vi "Config Scan Voltage.vi"(0 "VISA resource name":refnum<visa-resource-name>, 1 "Coupling (0)":i32 min=0 max=3, 2 "Floor (0.001)":dbl=0.001 min=0.0003 max=15.0, 3 "Ceiling (15)":dbl=15.0 min=0.0003 max=15.0, 4 "Method (discrete)":enum16{"discrete", "log10", "log2", "linear"}(ring), 5 "Method Value (1)":dbl=1.0 min=-100.0 max=100.0 format="%#_6f", 7 "error in":errorcluster) -> (20 "VISA resource name out":refnum<visa-resource-name>, 27 "error out":errorcluster)   [LabVIEW 2019, in "Andeen-Hagerling 2700(400 firmware).lvlib"]
doc: "Establishes the position of highest voltage scan within the multidimensional parameter scan system. Also sets the range of highest voltage parameter, Voltage, used during the scan as well as the direction in which the Voltage is changed each time a scan measurement is to be taken."
uses:
  Andeen-Hagerling 2700(400 firmware).lvlib
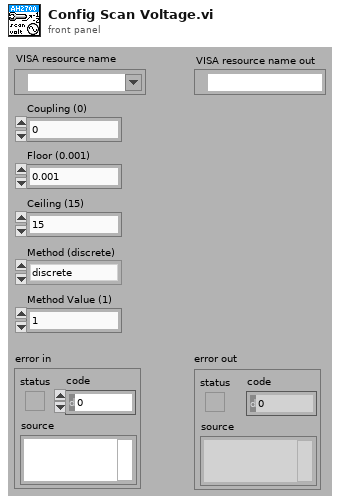
[diagram p1: front panel]
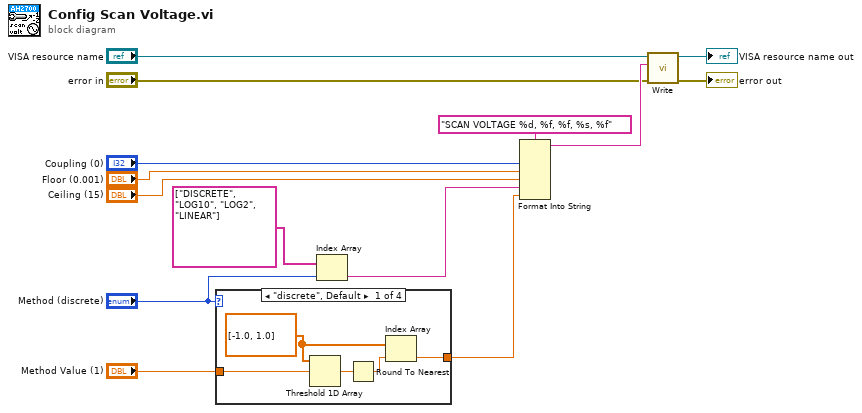
[diagram p0: block diagram]
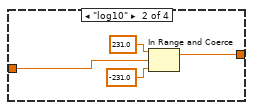
[diagram p2: hidden frame]
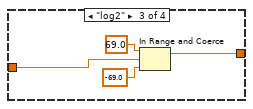
[diagram p3: hidden frame]
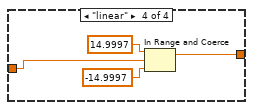
[diagram p4: hidden frame]
diagram:
  n1 = case shown="\"discrete\", Default" "Method (discrete)" {
    tunnel: "Method Value (1)" -> [w17 w20 w24 w28]
    tunnel: [w16 w21 w25 w29] -> w1
    frame "discrete", Default {
      w15 = dbl[] [-1.0, 1.0]
      n2 = Threshold 1D Array(2:w17, 3:w15) -> (0:w19:dbl)  [unwired: 1 in]
      n3 = Round To Nearest(number=w19) -> (nearest integer value=w18:dbl)
      n4 = Index Array(array=w15, index=w18) -> (element=w16:dbl)
    }
    frame "log10" {
      n5 = In Range and Coerce(upper limit=231.0, x=w20, lower limit=-231.0) -> (coerced(x)=w21:dbl)  [unwired: 1 out]
    }
    frame "log2" {
      n6 = In Range and Coerce(upper limit=69.0, x=w24, lower limit=-69.0) -> (coerced(x)=w25:dbl)  [unwired: 1 out]
    }
    frame "linear" {
      n7 = In Range and Coerce(upper limit=14.9997, x=w28, lower limit=-14.9997) -> (coerced(x)=w29:dbl)  [unwired: 1 out]
    }
  }
  n8 = Index Array(array=string[] ["DISCRETE", "LOG10", "LOG2", "LINEAR"], index="Method (discrete)") -> (element=w2:string)
  n9 = Format Into String(format string="SCAN VOLTAGE %d, %f, %f, %s, %f", "Coupling (0)", "Floor (0.001)", "Ceiling (15)", w2, w1) -> (resulting string=w12:string)  [unwired: 2 in, 1 out]
  n10 = call "Write.vi"("error in"="error in", "command"=w12, "VISA resource name"="VISA resource name") -> ("error out"=→"error out":errorcluster, "VISA resource name out"=→"VISA resource name out":refnum<visa-resource-name>)  [unwired: 7 in]
